vi "ATS_Trigger_4Ch.vi"(6 "ExtTrigControl":T1, 7 "Timeout (-1, Auto)":dbl=-1.0 format="%.2f", 8 "Engine Y":T4={"Source"=enum."Disable", "Slope"=enum."Positive", "Level"=128}, 9 "Engine X":T4={"Source"=enum."Chan_A", "Slope"=enum."Positive", "Level"=128}, 10 "TrigOperation":T6, 11 "DeviceIn":i32) -> (0 "Return Code":u32, 2 "Timeout":dbl format="%.2f", 3 "DeviceOut":i32)   [LabVIEW 2015]
doc: "_____AlazarTech, Scope_____\n\nSet the trigger parameters."
uses:
  ATS_ctl/ATS_TriggerEngine_4Ch.ctl
  ATS_ctl/ATS_TriggerSource_4Ch.ctl
  ATS_ctl/TriggerOperation.ctl
  ATS_ctl/ExtTrigger.ctl
  ATS_ctl/Coupling.ctl
  ATS_ctl/ExtTrigRange.ctl
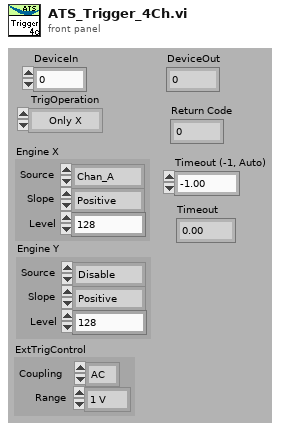
[diagram p1: front panel]
types:
  T1 = typedef "ExtTrigger.ctl" = cluster{"Coupling":T2, "Range":T3}
  T2 = typedef "Coupling.ctl" = enum16{"AC", "DC"}
  T3 = typedef "ExtTrigRange.ctl" = enum16{"1 V", "5 V", "TTL"}
  T4 = typedef "ATS_TriggerEngine_4Ch.ctl" = cluster{"Source":T5, "Slope":enum32{"Positive", "Negative"}, "Level":u32}
  T5 = typedef "ATS_TriggerSource_4Ch.ctl" = enum32{"Chan_A", "Chan_B", "External", "Disable", "Chan_C", "Chan_D"}
  T6 = typedef "TriggerOperation.ctl" = enum16{"Only X", "Only Y", "X or Y", "X and Y", "X xor Y", "X and not Y", "not X and Y"}
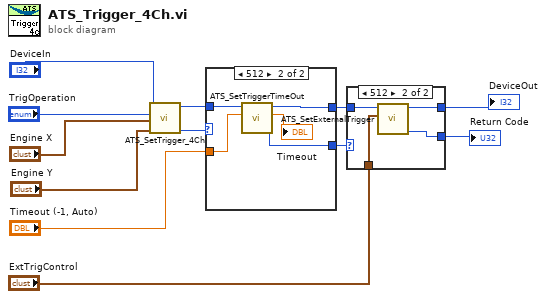
[diagram p0: block diagram]
diagram:
  n1 = call "ATS_SetTrigger_4Ch.vi"("Engine Y"="Engine Y", "Engine X"="Engine X", "TrigOperation"="TrigOperation", "DeviceIn"="DeviceIn") -> ("Return Code"=w9:u32, "DeviceOut"=w8:i32)  [unwired: 6 in]
  n2 = case shown="512" w9 {
    selector: w9 -> [w14 _]
    tunnel: w8 -> [w13 w19]
    tunnel: [w13 w18] -> w6
    tunnel: [w14 w17] -> w4
    tunnel: "Timeout (-1, Auto)" -> [_ w16]
    frame 0, Default {
    }
    frame 512 {
      n3 = call "ATS_SetTriggerTimeOut.vi"("Timeout (-1s)"=w16, "DeviceIn"=w19) -> ("Return Code"=w17:u32, "Timeout_Set"=→"Timeout":dbl, "DeviceOut"=w18:i32)  [unwired: 7 in]
    }
  }
  n4 = case shown="512" w4 {
    selector: w4 -> [w21 _]
    tunnel: w6 -> [w20 w25]
    tunnel: [w20 w24] -> w2
    tunnel: [w21 w23] -> w5
    tunnel: "ExtTrigControl" -> [_ w22]
    frame 0, Default {
    }
    frame 512 {
      n5 = call "ATS_SetExternalTrigger.vi"("ExtTrigControl"=w22, "DeviceIn"=w25) -> ("Return Code"=w23:u32, "DeviceOut"=w24:i32)  [unwired: 8 in]
    }
  }
  "Return Code" <- w5
  "DeviceOut" <- w2
